vi "T2_Test_Frequency_Calibration_V1.vi"() -> ()   [LabVIEW 2020]
uses:
  <instrlib>/niFgen/niFgen.llb/niFgen Output Mode.ctl
  <instrlib>/niFgen/niFgen.llb/niFgen Waveform Type.ctl
  <instrlib>/niFgen/niFgen.llb/niFgen_ctl Trigger DigEdge - Edge Values (Ring).ctl
  <instrlib>/niFgen/niFgen.llb/niFgen_ctl Trigger Source Values (Ring).ctl
  <instrlib>/niFgen/niFgen.llb/niFgen Trigger Mode.ctl
  <instrlib>/niScope/Controls/niScope acquisition type.ctl
  <instrlib>/niScope/Controls/niScope trigger slope.ctl
  <instrlib>/niScope/Controls/niScope trigger source.ctl
  <vilib>/Analysis/2dsp.llb/Integral Method.ctl
  <vilib>/Analysis/8numeric.llb/1D Numeric Integration.vi
  <vilib>/Utility/file.llb/Read Delimited Spreadsheet (DBL).vi
  <instrlib>/niFgen/niFgen.llb/niFgen Create Waveform (DBL).vi
  <instrlib>/niScope/Configure/Trigger/niScope Configure Trigger Edge.vi
  <instrlib>/niFgen/niFgen.llb/niFgen Configure Digital Edge Start Trigger.vi
  <instrlib>/niScope/Acquire/Fetch/niScope Fetch Cluster.vi
  <vilib>/Analysis/NI_AALPro.lvlib
panel:
  out "Frequency List (MHz)":dbl[](array[numeric])
  out "Power":dbl[](array[numeric])
  in  "Pulse Train File":path=path "C:/Users/localuser/OneDrive - University of South Carolina/NMR Research/Simulations/wfm.txt"
  in  "Starting Frequency":dbl=27440000.0 caption="Frequency" format="%.4p"
  out "Extracted T2 Decay - Current Scan":waveform(dbl)(graph)={"t0"=timestamp(0 s since 1904-01-01), "dt"=0.0025142857142857146, "Y"=array[865 elements]} caption="Waveform Graph"
  out "Scan Number":i32=1
  out "Pulse Echos - Current Scan":T1(graph) caption="Waveform Graph"
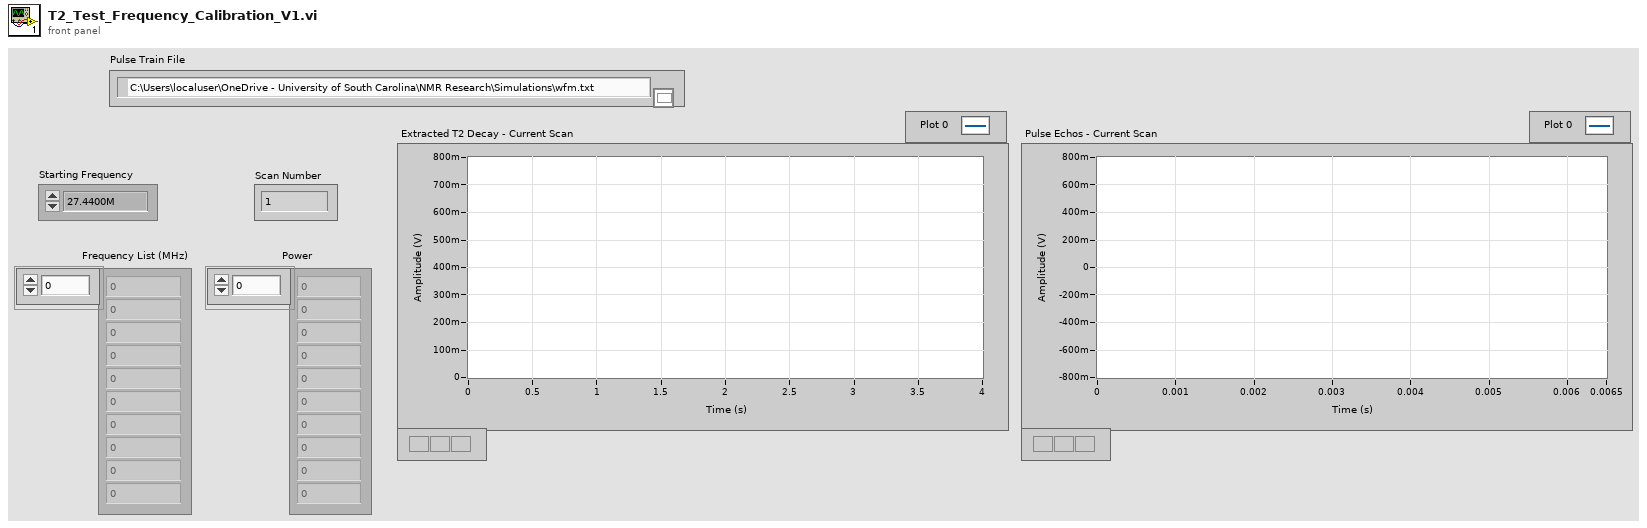
[diagram p1: front panel]
types:
  T1 = cluster{"relativeInitialX":dbl, "xIncrement":dbl, "wfm":dbl[]}
  T2 = typedef "niFgen Output Mode.ctl" = u32
  T3 = typedef "niScope trigger source.ctl" = string
  T4 = typedef "niFgen_ctl Trigger Source Values (Ring).ctl" = string
  T5 = typedef "NI_AALPro.lvlib/Integral Method.ctl" = i32
  T6 = typedef "niScope trigger slope.ctl" = i32
  T7 = typedef "niScope acquisition type.ctl" = i32
  T8 = typedef "niFgen Trigger Mode.ctl" = i32
  T9 = typedef "niFgen_ctl Trigger DigEdge - Edge Values (Ring).ctl" = i32
  T10 = typedef "niFgen Waveform Type.ctl" = i32
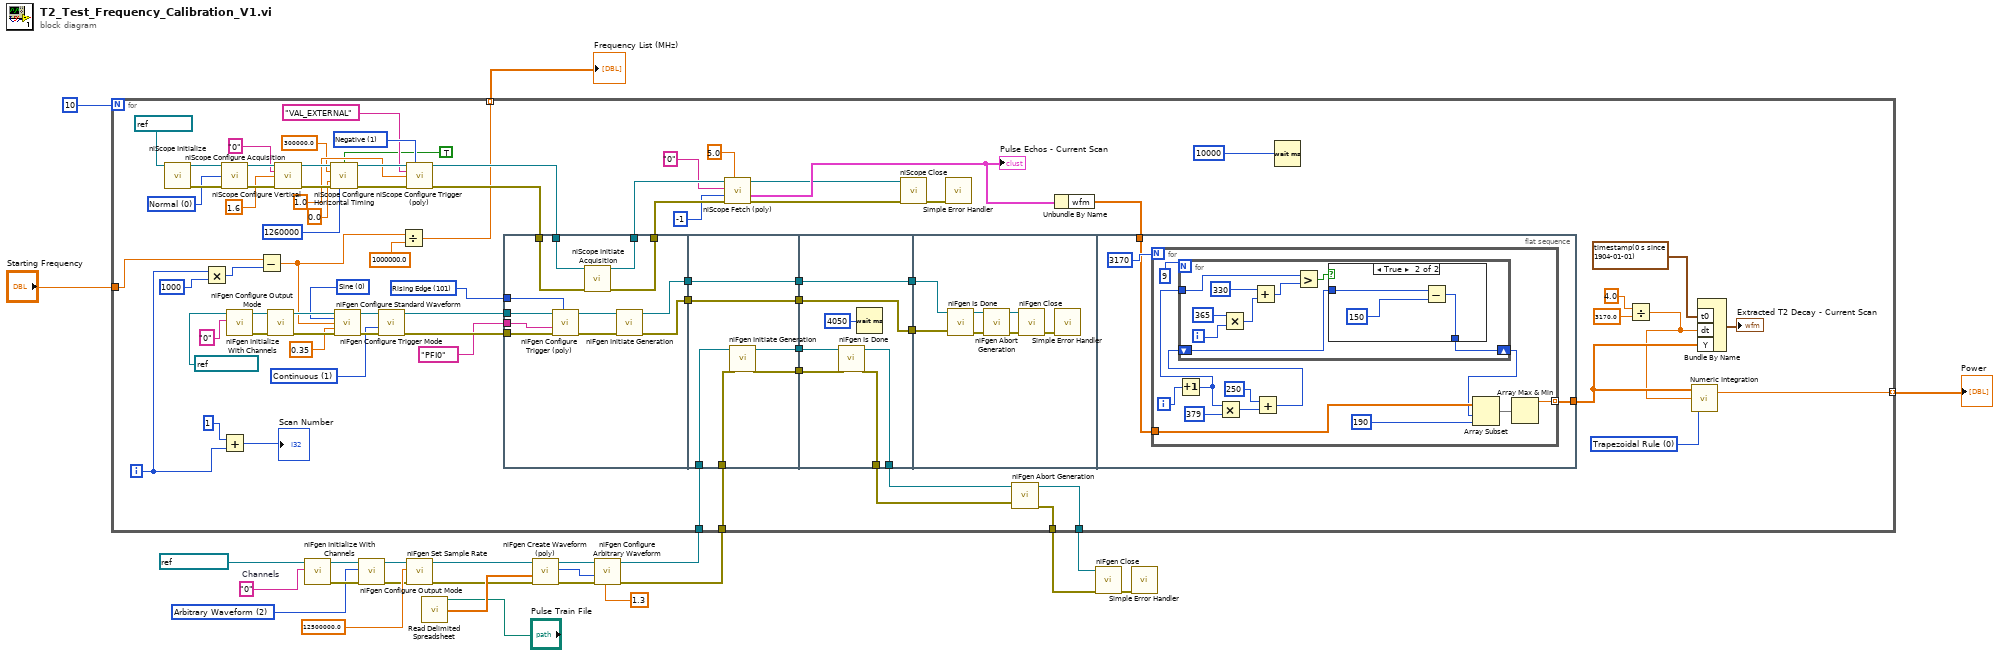
[diagram p0: block diagram]
diagram:
  w11 = "0"  # Channels
  w10 = T2 2 items=["Standard Function", "Frequency List", "Arbitrary Waveform", "Arbitrary Sequence", "Script"] ("output mode")
  n1 = call <instrlib>:"niFgen Initialize With Channels.vi"("Channel Name"=w11, "Resource Name"=refnum<k15> "PulseTrain" ("FGEN Resource Name 2")) -> ("error out"=w14:errorcluster, "Instrument Handle Out"=w15:refnum<k15>)  [unwired: 8 in]
  n2 = call <instrlib>:"niFgen Configure Output Mode.vi"("error in (no error)"=w14, "Output Mode (default: 0=Standard Function)"=w10, "Instrument Handle"=w15) -> ("error out"=w18:errorcluster, "Instrument Handle Out"=w17:refnum<k15>)  [unwired: 6 in]
  n3 = call <instrlib>:"niFgen Set Sample Rate.vi"("error in (no error)"=w18, "Sample Rate (Samp/s)"=12500000.0 ("Sample Rate"), "Instrument Handle"=w17) -> ("error out"=w21:errorcluster, "Instrument Handle Out"=w20:refnum<k15>)  [unwired: 7 in]
  n4 = call-poly <vilib>:"Read Delimited Spreadsheet.vi"("file path (dialog if empty)"="Pulse Train File") -> ("first row"=w22:dbl[])  [unwired: 9 in, 5 out]
  n5 = call-poly <instrlib>:"niFgen Create Waveform (poly).vi"("error in (no error)"=w21, "Waveform Data Array"=w22, "Instrument Handle"=w20) -> ("error out"=w24:errorcluster, "Waveform Handle"=w25:i32, "Instrument Handle Out"=w23:refnum<k15>)  [unwired: 6 in]
  n6 = call <instrlib>:"niFgen Configure Arbitrary Waveform.vi"("Gain"=1.3, "error in (no error)"=w24, "Waveform Handle"=w25, "Instrument Handle"=w23) -> ("error out"=w9:errorcluster, "Instrument Handle Out"=w8:refnum<k15>)  [unwired: 6 in]
  n7 = for {
    N: 10 ("Number of Scans") -> [_]
    tunnel: w9 -> [w86]
    tunnel: w8 -> [w85]
    tunnel: [w84] -> w6
    tunnel: [w83] -> w5
    tunnel: [w33] -> w3 mode=indexing
    tunnel: "Starting Frequency" -> [w32]
    tunnel: [w28] -> w1 mode=indexing
    i -> [w31]
    w42 = T5 0 items=["Trapezoidal Rule", "Simpson's Rule", "Simpson's 3/8 Rule", "Bode Rule"] ("integration method")
    w71 = T6 1 items=["Positive", "Negative"] ("trigger slope")
    w72 = T7 0 items=["Normal"=0, "Flex Res"=1, "DDC"=3] ("acquisition Type")
    w90 = T8 1 items=["Single", "Continuous", "Stepped", "Burst"] ("Trigger Mode (default: 1=continuous)")
    w94 = T9 101 items=["Rising Edge"=101, "Falling Edge"=102] ("Edge (Rising)")
    w95 = T10 0 items=["Sine", "Square", "Triangle", "Ramp Up", "Ramp Down", "DC", "Noise", "User"] ("Waveform")
    n8 = call <instrlib>:"niScope Initialize.vi"("resource name"=refnum<k15> "OScope") -> ("instrument handle"=w73:refnum<k15>, "error out"=w74:errorcluster)  [unwired: 13 in]
    n9 = Multiply(x=w31, y=1000) -> (x*y=w29:i32)
    n10 = call <instrlib>:"niScope Configure Acquisition.vi"("instrument handle"=w73, "acquisition Type"=w72, "error in"=w74) -> ("instrument handle out"=w76:refnum<k15>, "error out"=w77:errorcluster)  [unwired: 11 in]
    n11 = Add(x=1, y=w31) -> (x+y=→"Scan Number":i32)
    n12 = call <instrlib>:"niFgen Initialize With Channels.vi"("Channel Name"="0", "Resource Name"=refnum<k15> "FuncGen" ("Sine Wave Module")) -> ("error out"=w100:errorcluster, "Instrument Handle Out"=w103:refnum<k15>)  [unwired: 8 in]
    n13 = Subtract(x=w32, y=w29) -> (x-y=w27:dbl)
    n14 = call <instrlib>:"niFgen Configure Output Mode.vi"("error in (no error)"=w100, "Instrument Handle"=w103) -> ("error out"=w99:errorcluster, "Instrument Handle Out"=w102:refnum<k15>)  [unwired: 7 in]
    n15 = call <instrlib>:"niScope Configure Vertical.vi"("instrument handle"=w76, "channels"="0", "vertical range"=1.6, "error in"=w77) -> ("instrument handle out"=w78:refnum<k15>, "error out"=w79:errorcluster)  [unwired: 10 in]
    n16 = call <instrlib>:"niScope Configure Horizontal Timing.vi"("instrument handle"=w78, "enforce realtime"=TRUE, "min sample rate"=300000.0, "reference position"=0.0, "error in"=w79, "min record length"=1260000) -> ("instrument handle out"=w80:refnum<k15>, "error out"=w81:errorcluster)  [unwired: 8 in]
    n17 = call <instrlib>:"niFgen Configure Standard Waveform.vi"("Instrument Handle"=w102, "Waveform"=w95, "Frequency"=w27, "Amplitude"=0.35, "error in (no error)"=w99) -> ("Instrument Handle Out"=w101:refnum<k15>, "error out"=w98:errorcluster)  [unwired: 9 in]
    n18 = call <instrlib>:"niFgen Configure Trigger Mode.vi"("error in (no error)"=w98, "Trigger Mode (default: 1=continuous)"=w90, "Instrument Handle"=w101) -> ("error out"=w93:errorcluster, "Instrument Handle Out"=w91:refnum<k15>)  [unwired: 7 in]
    n19 = Divide(x=w27, y=1000000.0) -> (x/y=w28:dbl)
    n20 = call-poly <instrlib>:"niScope Configure Trigger (poly).vi"("instrument handle"=w80, "trigger slope"=w71, "trigger source"=T3 "VAL_EXTERNAL", "trigger level"=1.0, "error in"=w81) -> ("instrument handle out"=w65:refnum<k15>, "error out"=w64:errorcluster)  [unwired: 9 in]
    n21 = flat-sequence {
      tunnel: w94 -> [w114]
      tunnel: w93 -> [w113]
      tunnel: T4 "PFI0" ("Source") -> [w112]
      tunnel: w91 -> [w111]
      tunnel: w65 -> [w109]
      tunnel: w64 -> [w108]
      tunnel: [w107] -> w63
      tunnel: [w106] -> w62
      tunnel: [w105] -> w52
      tunnel: [w104] -> w49
      tunnel: w86 -> [w121]
      tunnel: w85 -> [w120]
      tunnel: [w119] -> w56
      tunnel: [w118] -> w55
      tunnel: [w117] -> w53
      tunnel: w52 -> [w117]
      tunnel: [w116] -> w50
      tunnel: w49 -> [w116]
      tunnel: [w127] -> w88
      tunnel: [w126] -> w87
      tunnel: w56 -> [w125]
      tunnel: w55 -> [w124]
      tunnel: [w123] -> w54
      tunnel: w53 -> [w123]
      tunnel: [w122] -> w51
      tunnel: w50 -> [w122]
      tunnel: w54 -> [w130]
      tunnel: w51 -> [w129]
      tunnel: w39 -> [w137]
      tunnel: [w136] -> w44
      frame #0 {
        n22 = call-poly <instrlib>:"niFgen Configure Trigger (poly).vi"("Edge (Rising)"=w114, "error in (no error)"=w113, "Source"=w112, "Instrument Handle"=w111) -> ("error out"=w110:errorcluster, "Instrument Handle Out"=w115:refnum<k15>)  [unwired: 6 in]
        n23 = call <instrlib>:"niScope Initiate Acquisition.vi"("instrument handle"=w109, "error in"=w108) -> ("instrument handle out"=w107:refnum<k15>, "error out"=w106:errorcluster)  [unwired: 12 in]
        n24 = call <instrlib>:"niFgen Initiate Generation.vi"("error in (no error)"=w110, "Instrument Handle"=w115) -> ("error out"=w104:errorcluster, "Instrument Handle Out"=w105:refnum<k15>)  [unwired: 8 in]
      }
      frame #1 {
        n25 = call <instrlib>:"niFgen Initiate Generation.vi"("error in (no error)"=w121, "Instrument Handle"=w120) -> ("error out"=w118:errorcluster, "Instrument Handle Out"=w119:refnum<k15>)  [unwired: 8 in]
      }
      frame #2 {
        n26 = call <instrlib>:"niFgen Is Done.vi"("error in (no error)"=w124, "Instrument Handle"=w125) -> ("error out"=w127:errorcluster, "Instrument Handle Out"=w126:refnum<k15>)  [unwired: 7 in, 1 out]
        n27 = Wait (ms)(milliseconds to wait=u32 4050) -> ()  [unwired: 1 out]
      }
      frame #3 {
        n28 = call <instrlib>:"niFgen Is Done.vi"("error in (no error)"=w129, "Instrument Handle"=w130) -> ("error out"=w133:errorcluster, "Instrument Handle Out"=w132:refnum<k15>)  [unwired: 7 in, 1 out]
        n29 = call <instrlib>:"niFgen Abort Generation.vi"("error in (no error)"=w133, "Instrument Handle"=w132) -> ("error out"=w134:errorcluster, "Instrument Handle Out"=w135:refnum<k15>)  [unwired: 8 in]
        n30 = call <instrlib>:"niFgen Close.vi"("error in (no error)"=w134, "Instrument Handle"=w135) -> ("error out"=w131:errorcluster)  [unwired: 9 in]
        n31 = call <vilib>:"Simple Error Handler.vi"("error in (no error)"=w131) -> ()  [unwired: 4 in, 5 out]
      }
      frame #4 {
        n32 = for {
          N: 3170 -> [_]
          tunnel: [w148] -> w136 mode=indexing
          tunnel: w137 -> [w147]
          i -> [w140]
          n33 = Increment(x=w140) -> (x+1=w139:i32)
          n34 = Multiply(x=w139, y=379) -> (x*y=w146:i32)
          n35 = Add(x=250, y=w146) -> (x+y=w142:i32)
          n36 = for {
            N: 9 -> [_]
            tunnel: w139 -> [w159]
            shift-right: [w152] -> w141
            shift-left: w142 -> [w153]
            i -> [w151]
            n37 = Multiply(x=365, y=w151) -> (x*y=w155:i32)
            n38 = Add(x=330, y=w155) -> (x+y=w157:i32)
            n39 = Greater?(x=w159, y=w157) -> (0:w154:bool)
            n40 = case shown="True" w154 {
              tunnel: w153 -> [w160 w163]
              tunnel: [w160 w162] -> w152
              frame False {
              }
              frame True {
                n41 = Subtract(x=w163, y=150) -> (x-y=w162:i32)
              }
            }
          }
          n42 = Array Subset(array=w147, index=w141, length=190 ("y")) -> (w149:dbl[])
          n43 = Array Max & Min(array=w149) -> (max value=w148:dbl)  [unwired: 3 out]
        }
      }
    }
    n44 = call-poly <instrlib>:"niScope Fetch (poly).vi"("timeout"=5.0, "error in"=w62, "numSamples"=-1, "channels"="0", "instrument handle"=w63) -> ("error out"=w35:errorcluster, "waveform"=w38:T1, "instrument handle out"=w36:refnum<k15>)  [unwired: 3 in, 1 out]
    "Pulse Echos - Current Scan" <- w38
    n45 = call <instrlib>:"niScope Close.vi"("instrument handle"=w36, "error in"=w35) -> ("error out"=w82:errorcluster)  [unwired: 13 in]
    n46 = call <vilib>:"Simple Error Handler.vi"("error in (no error)"=w82) -> ()  [unwired: 4 in, 5 out]
    n47 = call <instrlib>:"niFgen Abort Generation.vi"("error in (no error)"=w88, "Instrument Handle"=w87) -> ("error out"=w84:errorcluster, "Instrument Handle Out"=w83:refnum<k15>)  [unwired: 8 in]
    n48 = Unbundle By Name(w38) -> ("wfm"=w39:dbl[])
    n49 = Wait (ms)(milliseconds to wait=u32 10000 ("Delay Time (ms)")) -> ()  [unwired: 1 out]
    n50 = Divide(x=4.0, y=3170.0) -> (x/y=w43:dbl)
    n51 = call-poly <vilib>:"Numeric Integration.vi"("integration method"=w42, "dt"=w43, "Input Array"=w44) -> ("result"=w33:dbl)  [unwired: 1 out]
    n52 = Bundle By Name("t0"=timestamp(0 s since 1904-01-01), "dt"=w43, "Y"=w44) -> (→"Extracted T2 Decay - Current Scan":waveform(dbl))  [unwired: 1 in]
  }
  "Power" <- w3
  "Frequency List (MHz)" <- w1
  n53 = call <instrlib>:"niFgen Close.vi"("error in (no error)"=w6, "Instrument Handle"=w5) -> ("error out"=w7:errorcluster)  [unwired: 9 in]
  n54 = call <vilib>:"Simple Error Handler.vi"("error in (no error)"=w7) -> ()  [unwired: 4 in, 5 out]
